vi "Date n Time.vi"() -> (1 "Date & Time":string)   [LabVIEW 2026, in "TALOS.lvlib"]
doc: "This VI returns a string with the current date and time. Useful to be sure to use the same format in all the VIs."
uses:
  TALOS.lvlib
panel:
  # "NOTE: if you modify this VI, check that the Log.lvclass->Rotate still works!"
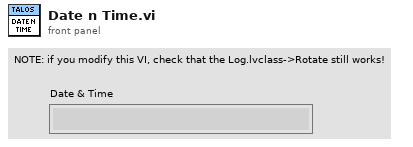
[diagram p1: front panel]
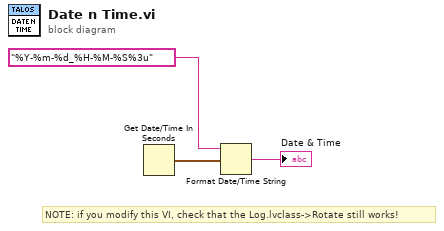
[diagram p0: block diagram]
diagram:
  # "NOTE: if you modify this VI, check that the Log.lvclass->Rotate still works!"
  n1 = Get Date/Time In Seconds() -> (seconds since 1Jan1904=w2:timestamp)
  n2 = Format Date/Time String(time format string (%c)="%Y-%m-%d_%H-%M-%S%3u", seconds (now)=w2) -> (date/time string=→"Date & Time":string)  [unwired: 1 in]
